vi "Test RunTime.vi"() -> ()   [LabVIEW 2020]
uses:
  Typdefs/Cluster Test.ctl
  Typdefs/Enum Test.ctl
  Library/Typedefs/Cluster Test.ctl
  Library/Typedefs/Enum Test.ctl
  Class/Typedefs/Cluster Test.ctl
  Class/Typedefs/Enum Test.ctl
  Class/Test Class.lvclass
  Library/Test Class/Test Class.lvclass
  Library/Test Class/Typedefs/Cluster Test.ctl
  Library/Test Class/Typedefs/Enum Test.ctl
  Library/Test Library.lvlib
panel:
  in  "Library.Class.TypeDef:Cluster 2":T1
  in  "Class.TypeDef:Cluster 2":T2
  in  "Test Library.lvlib:Test Class.lvclass 2":refnum<class "Test Class.lvclass">
  in  "Test Class.lvclass 2":refnum<class "Test Class.lvclass">
  in  "Library.TypeDef:Cluster 2":T3
  in  "TypeDef:Cluster 2":T4
  in  "Refresh Menus":bool
  in  "Checkbox":bool
  out "Numeric":i32
  out "Library.Class.TypeDef:Enum":T5
  out "Library.Class.TypeDef:Cluster":T1
  out "Test Library.lvlib:Test Class.lvclass":refnum<class "Test Class.lvclass">
  out "Test Class.lvclass":refnum<class "Test Class.lvclass">
  out "Class.TypeDef:Enum":T6
  out "Class.TypeDef:Cluster":T2
  out "Library.TypeDef:Enum":T7
  out "Library.TypeDef:Cluster":T3
  out "TypeDef:Enum":T8
  out "TypeDef:Cluster":T4
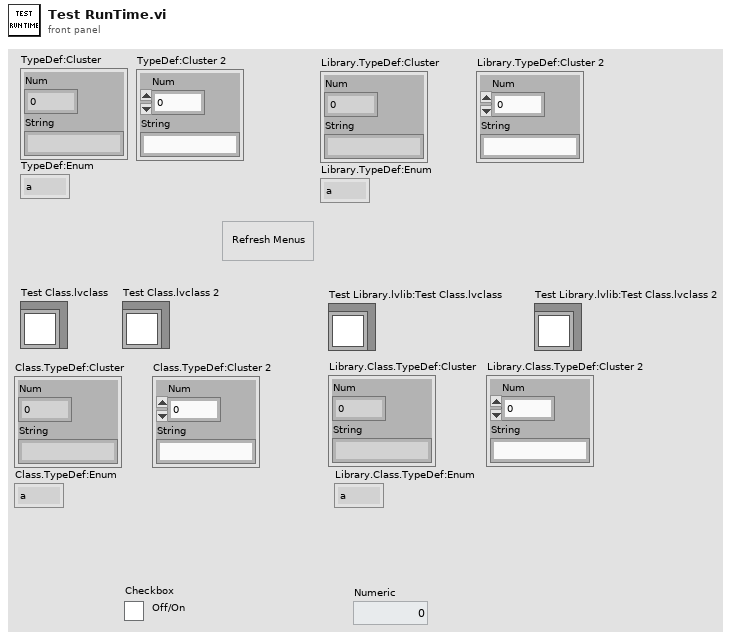
[diagram p1: front panel]
types:
  T1 = typedef "Test Library.lvlib/Test Class.lvclass/Cluster Test.ctl" = cluster{"Num":i32, "String":string}
  T2 = typedef "Test Class.lvclass/Cluster Test.ctl" = cluster{"Num":i32, "String":string}
  T3 = typedef "Test Library.lvlib/Cluster Test.ctl" = cluster{"Num":i32, "String":string}
  T4 = typedef "Cluster Test.ctl" = cluster{"Num":i32, "String":string}
  T5 = typedef "Test Library.lvlib/Test Class.lvclass/Enum Test.ctl" = enum16{"a", "b"}
  T6 = typedef "Test Class.lvclass/Enum Test.ctl" = enum16{"a", "b"}
  T7 = typedef "Test Library.lvlib/Enum Test.ctl" = enum16{"a", "b"}
  T8 = typedef "Enum Test.ctl" = enum16{"a", "b"}
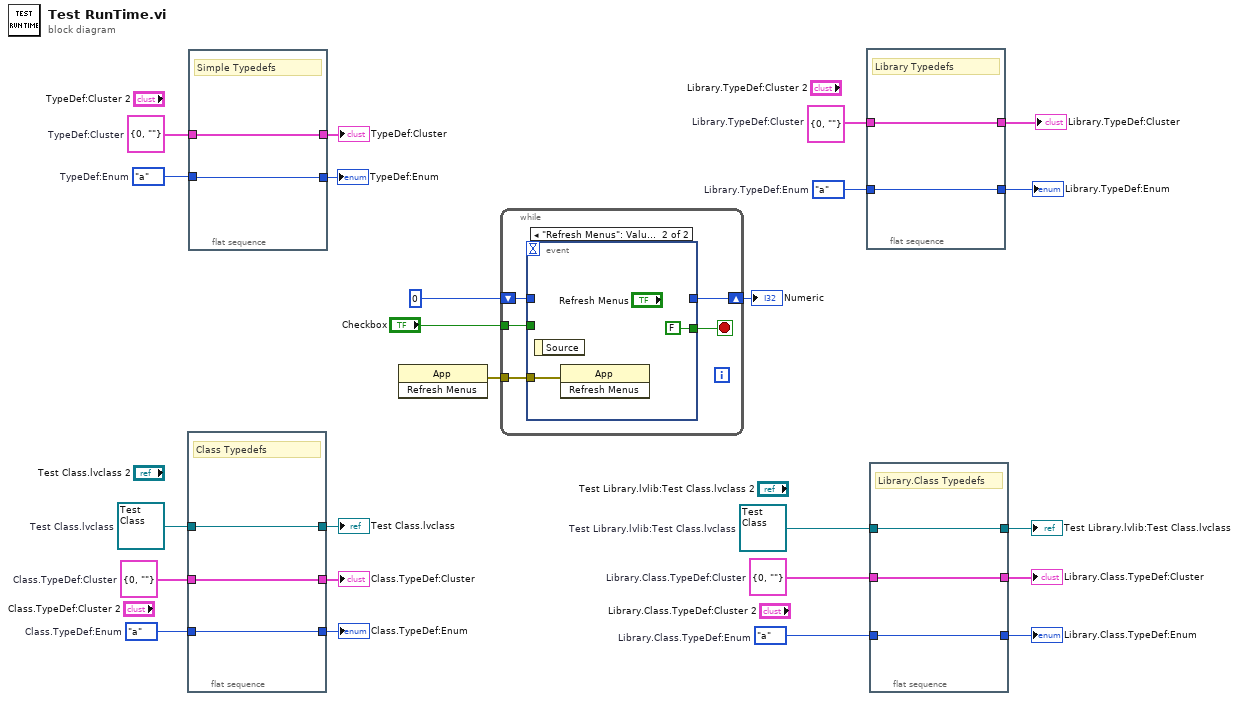
[diagram p0: block diagram]
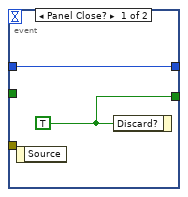
[diagram p2: hidden frame]
diagram:
  w8 = refnum<class "Test Class.lvclass"> refnum  # Test Library.lvlib:Test Class.lvclass
  w4 = Enum_Test."a"  # Library.Class.TypeDef:Enum
  w6 = T1 {"Num"=0, "String"=""}  # Library.Class.TypeDef:Cluster
  w10 = refnum<class "Test Class.lvclass"> refnum  # Test Class.lvclass
  w12 = Enum_Test."a"  # Class.TypeDef:Enum
  w14 = T2 {"Num"=0, "String"=""}  # Class.TypeDef:Cluster
  w16 = Enum_Test."a"  # Library.TypeDef:Enum
  w18 = T3 {"Num"=0, "String"=""}  # Library.TypeDef:Cluster
  w22 = T4 {"Num"=0, "String"=""}  # TypeDef:Cluster
  w20 = Enum_Test."a"  # TypeDef:Enum
  n1 = flat-sequence {
    tunnel: [w27] -> w15
    tunnel: w14 -> [w27]
    tunnel: [w26] -> w13
    tunnel: w12 -> [w26]
    tunnel: [w25] -> w11
    tunnel: w10 -> [w25]
    frame #0 {
      # "Class Typedefs"
    }
  }
  n2 = flat-sequence {
    tunnel: [w29] -> w23
    tunnel: w22 -> [w29]
    tunnel: [w28] -> w21
    tunnel: w20 -> [w28]
    frame #0 {
      # "Simple Typedefs"
    }
  }
  n3 = invoke class="App" method="Refresh Menus"() -> (error out=w24:errorcluster)  [unwired: 3 in, 2 out]
  n4 = while {
    tunnel: w24 -> [w34]
    tunnel: "Checkbox" -> [w31]
    shift-right: [w33] -> w3
    shift-left: 0 -> [w32]
    stop <- w30 stop-if-true
    n5 = event shown="[1] \"Refresh Menus\": Value Change" {
      selector: _ -> [_ _]
      dyn-events: _ -> [_ _]
      timeout: _ -> [_ _]
      tunnel: w34 -> [_ w37]
      tunnel: [w36 _] -> w33
      tunnel: w32 -> [w36 _]
      tunnel: w31 -> [_ _]
      tunnel: [w35 FALSE ("Discard?")] -> w30
      event Panel Close? {
        w35 = TRUE ("Discard?")
        n6 = event-data() -> ()  [unwired: 1 in, 1 out]
        n7 = event-data("Discard?"=w35) -> ()  [unwired: 1 in, 1 out]
      }
      event "Refresh Menus": Value Change {
        n8 = event-data() -> ()  [unwired: 1 in, 1 out]
        n9 = invoke class="App" method="Refresh Menus"(error in=w37) -> ()  [unwired: 2 in, 3 out]
      }
    }
  }
  "Numeric" <- w3
  n10 = flat-sequence {
    tunnel: [w40] -> w19
    tunnel: w18 -> [w40]
    tunnel: [w39] -> w17
    tunnel: w16 -> [w39]
    frame #0 {
      # "Library Typedefs"
    }
  }
  n11 = flat-sequence {
    tunnel: [w43] -> w9
    tunnel: w8 -> [w43]
    tunnel: [w42] -> w7
    tunnel: w6 -> [w42]
    tunnel: [w41] -> w5
    tunnel: w4 -> [w41]
    frame #0 {
      # "Library.Class Typedefs"
    }
  }
  "TypeDef:Cluster" <- w23
  "TypeDef:Enum" <- w21
  "Library.TypeDef:Cluster" <- w19
  "Library.TypeDef:Enum" <- w17
  "Class.TypeDef:Cluster" <- w15
  "Class.TypeDef:Enum" <- w13
  "Test Class.lvclass" <- w11
  "Test Library.lvlib:Test Class.lvclass" <- w9
  "Library.Class.TypeDef:Cluster" <- w7
  "Library.Class.TypeDef:Enum" <- w5
